vi "Switch inputs if vertical.vi"(9 "Y length":dbl, 11 "X length":dbl) -> (0 "Vertical":bool, 1 "Number of lines":dbl, 3 "Length":dbl)   [LabVIEW 2013]
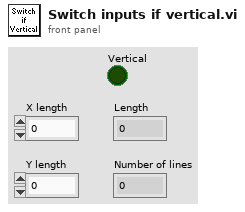
[diagram p1: front panel]
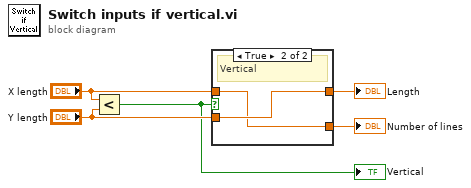
[diagram p0: block diagram]
diagram:
  n1 = Less?(x="X length", y="Y length") -> (x < y?=w1:bool)
  "Vertical" <- w1
  n2 = case shown="True" w1 {
    tunnel: "X length" -> [w7 w8]
    tunnel: "Y length" -> [w6 w9]
    tunnel: [w7 w9] -> w5
    tunnel: [w6 w8] -> w4
    frame False {
      # "Horisontal"
    }
    frame True {
      # "Vertical"
    }
  }
  "Length" <- w5
  "Number of lines" <- w4
